vi "UpVisionGlb.vi"() -> ()   [LabVIEW 2019]
panel:
  in  "Up Change Exposure":refnum<vi>
  in  "UpCamCenter":cluster{"X":dbl, "Y":dbl}
  in  "UpAngle":dbl
  in  "Upscale":dbl
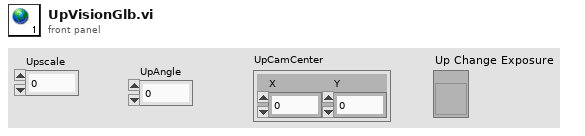
[diagram p1: front panel]
diagram:
